vi "stop.vi"(0 "Dataflow In":errorcluster, 1 "Stop In":refnum<vi>) -> (2 "Stop Out":bool, 5 "Dataflow Out":errorcluster)   [LabVIEW 2019]
uses:
  lib/libSimulationControl/libSimulationControl.lvlib
panel:
  # "*******************************************************************\nBiogas Plant Control\n\nAuthor: Paul Zügel\nGCSC-Frankfurt am Main 2020\n\n*******************************************************************"
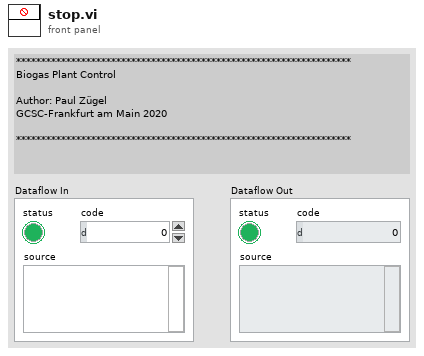
[diagram p1: front panel]
types:
  T1 = enum32{"Invalid", "Standard", "Closed", "Hidden", "Minimized", "Maximized"}
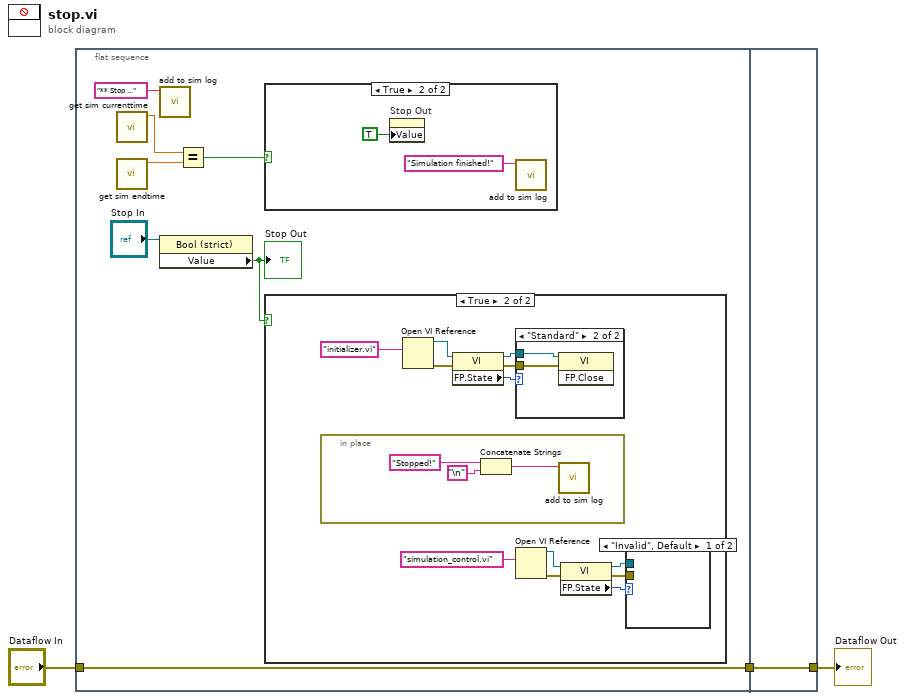
[diagram p0: block diagram]
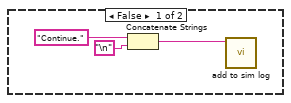
[diagram p3: hidden frame]
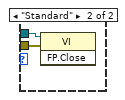
[diagram p5: hidden frame]
diagram:
  n1 = flat-sequence {
    tunnel: "Dataflow In" -> [w8]
    tunnel: [w8] -> w2
    tunnel: w2 -> [w35]
    tunnel: [w35] -> w1
    frame #0 {
      n2 = call "get sim currenttime.vi"() -> ("function return"=w4:dbl)  [unwired: 10 in, 1 out]
      n3 = call "get sim endtime.vi"() -> ("function return"=w5:dbl)  [unwired: 10 in, 1 out]
      n4 = call "add to sim log.vi"("log"="** Stop ..." ("string")) -> ()  [unwired: 10 in, 1 out]
      n5 = property on="Property Node" class="Bool (strict)"(reference="Stop In") -> ("Value"=w9:bool)  [unwired: 1 in, 2 out]
      "Stop Out" <- w9
      n6 = Equal?(x=w4, y=w5) -> (x = y?=w6:bool)
      n7 = case shown="True" w6 {
        frame False {
        }
        frame True {
          n8 = property on="Stop Out" class="Bool (strict)"("Value"=TRUE ("Stop Button")) -> ()  [unwired: 2 in, 2 out]
          n9 = call "add to sim log.vi"("log"="Simulation finished!") -> ()  [unwired: 10 in, 1 out]
        }
      }
      n10 = case shown="True" w9 {
        frame False {
          n11 = Concatenate Strings("Continue." ("string"), "\n") -> (w15:string)
          n12 = call "add to sim log.vi"("log"=w15) -> ()  [unwired: 10 in, 1 out]
        }
        frame True {
          n13 = in-place {
            n14 = Concatenate Strings("Stopped!" ("string"), "\n") -> (w28:string)
            n15 = call "add to sim log.vi"("log"=w28) -> ()  [unwired: 10 in, 1 out]
          }
          n16 = Open VI Reference(vi path="initializer.vi") -> (vi reference=w17:refnum<vi>, error out=w16:errorcluster)  [unwired: 5 in]
          n17 = property class="VI"(reference=w17, error in=w16) -> (reference out=w19:refnum<vi>, error out=w18:errorcluster, "FP.State"=w20:T1)
          n18 = case shown="\"Standard\"" w20 {
            tunnel: w19 -> [_ w32]
            tunnel: w18 -> [_ w31]
            frame "Invalid", Default {
            }
            frame "Standard" {
              n19 = invoke class="VI" method="FP.Close"(reference=w32, error in=w31) -> ()  [unwired: 1 in, 3 out]
            }
          }
          n20 = Open VI Reference(vi path="simulation_control.vi") -> (vi reference=w22:refnum<vi>, error out=w21:errorcluster)  [unwired: 5 in]
          n21 = property class="VI"(reference=w22, error in=w21) -> (reference out=w24:refnum<vi>, error out=w23:errorcluster, "FP.State"=w25:T1)
          n22 = case shown="\"Invalid\", Default" w25 {
            tunnel: w24 -> [_ w34]
            tunnel: w23 -> [_ w33]
            frame "Invalid", Default {
            }
            frame "Standard" {
              n23 = invoke class="VI" method="FP.Close"(reference=w34, error in=w33) -> ()  [unwired: 1 in, 3 out]
            }
          }
        }
      }
    }
    frame #1 {
    }
  }
  "Dataflow Out" <- w1
